vi "PR4000 cfg slave value.vi"(8 "error in (no error)":errorcluster, 10 "Channel parsed command info":T1, 11 "MKS4000b in":refnum<class "ISSI_Iris.lvclass">) -> (0 "error out":errorcluster, 2 "new commands":string, 3 "MKS4000b out":refnum<class "ISSI_Iris.lvclass">)   [LabVIEW 2020]
uses:
  shared/CompressAndUpdate(Poly)/CompressAndUpdate(Numeric).vi
  ISSI_Iris.lvclass
  C:/GEECS/Developers Version/source/Device Drivers/BaseDriver/BaseDriver.lvclass
  C:/GEECS/Developers Version/source/Device Drivers/ISSI_Iris/ISSI_Iris.lvclass
  Shared/Device Driver/channel parsed cmd cluster.ctl
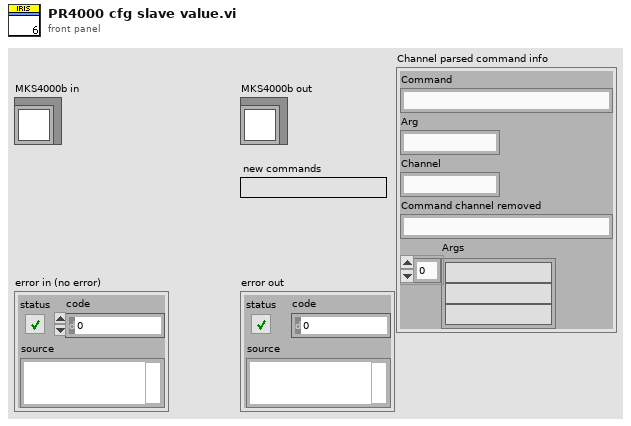
[diagram p1: front panel]
types:
  T1 = typedef "channel parsed cmd cluster.ctl" = cluster{"Command":string, "Arg":string, "Channel":string, "Command channel removed":string, "Args":string[]}
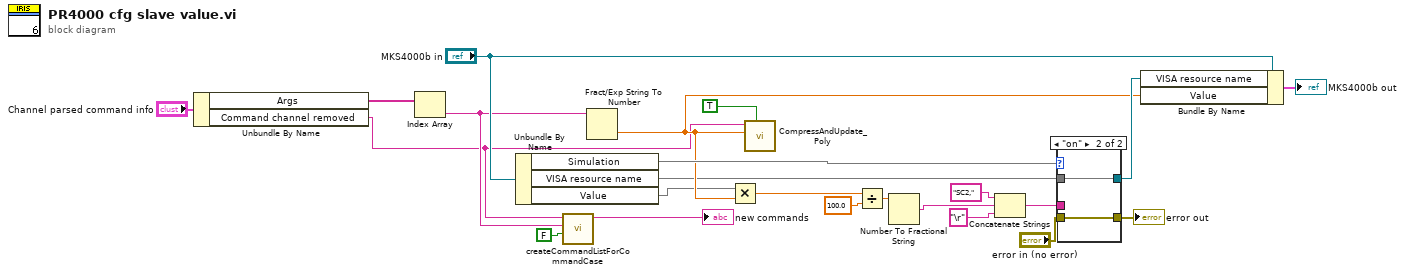
[diagram p0: block diagram]
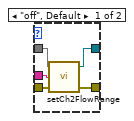
[diagram p2: hidden frame]
diagram:
  n1 = Unbundle By Name("Channel parsed command info") -> ("Args"=w2:string[], "Command channel removed"=w1:string)
  n2 = Index Array(array=w2) -> (element=w6:string)  [unwired: 1 in]
  n3 = Unbundle By Name("MKS4000b in") -> ("Simulation"=w23, "VISA resource name"=w10, "Value"=w8)
  n4 = call "createCommandListForCommandCase.vi"("immediate Check (only once)"=FALSE, "setvalue"=w6, "command"=w1) -> ("new commands"=→"new commands":string)  [unwired: 8 in]
  n5 = Fract/Exp String To Number(string=w6) -> (number=w12:dbl)  [unwired: 3 in, 1 out]
  n6 = Multiply(x=w8, y=w12) -> (x*y=w14:dbl)
  n7 = call-poly "CompressAndUpdate_Poly.vi"("force CVT update (false)"=TRUE ("force CVT update"), "Numeric"=w12, "command or variable name"=w1) -> ()  [unwired: 8 in, 1 out]
  n8 = Divide(x=w14, y=100.0) -> (x/y=w19:dbl)
  n9 = Number To Fractional String(number=w19) -> (F-format string=w20:string)  [unwired: 3 in]
  n10 = Concatenate Strings("SC2," ("string"), w20, "\r" ("string")) -> (w17:string)
  n11 = case shown="\"on\"" w23 {
    tunnel: "error in (no error)" -> [w28 w29]
    tunnel: w10 -> [w27 w30]
    tunnel: [w26 w29] -> w11
    tunnel: w17 -> [w25 _]
    tunnel: [w24 w30] -> w21
    frame "off", Default {
      n12 = call "setCh2FlowRange.vi"("error"=w28, "command in"=w25, "Comport PR4000"=w27) -> ("error out"=w26:errorcluster, "VISA resource name out"=w24:refnum<visa-resource-name>)  [unwired: 1 out]
    }
    frame "on" {
    }
  }
  "error out" <- w11
  n13 = Bundle By Name(cluster="MKS4000b in", "VISA resource name"=w21, "Value"=w12) -> (→"MKS4000b out":cluster{})
